vi "InitMessageBroker.vi"(8 "error in (no error)":errorcluster, 10 "Topic Actor":refnum<class "Topic Actor.lvclass">, 11 "Broker Name":string) -> (0 "error out":errorcluster, 3 "Message Broker Ref":refnum<data-value>)   [LabVIEW 2016, in "Stream Mediator.lvlib" / "Message Broker.lvclass"]
doc: "--\nCopyright © 2017 Composed SystemsI All rights reserved.\n\nAuthor: Jon McBee <jon.mcbee@composed.io>\n\nThis library is provided \"AS IS\" ,WITHOUT WARRANTIES OR\nCONDITIONS OF ANY KIND, either express or implied.\n\nComposed Systems -- composed.io\n\nStream 0.0.1.1\nJon McBee - Composed Systems\nCopyright (c) 2017, Composed Systems"
uses:
  <userlib>/Composed Systems/Stream/Mediator/Classes/Message Broker/Message Broker.lvclass
  <userlib>/Composed Systems/Stream/Mediator/Classes/Topic Actor/Topic Actor.lvclass
  <userlib>/Composed Systems/Stream/Mediator/Classes/Topic Actor Look Up Table/Topic Actor Look Up Table.lvclass
  <userlib>/Composed Systems/Stream/Mediator/Classes/Message Broker/Message Broker.lvclass/Message Broker.ctl
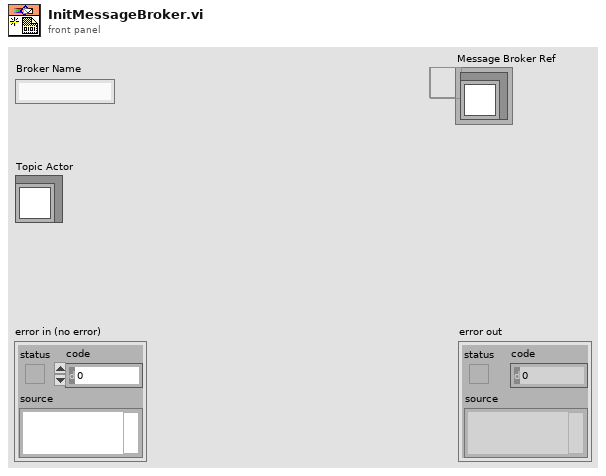
[diagram p1: front panel]
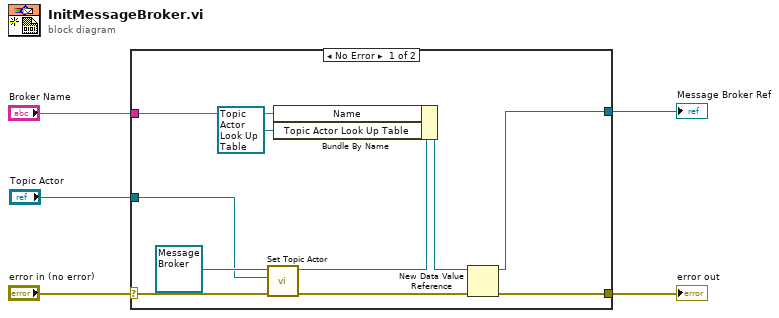
[diagram p0: block diagram]
diagram:
  n1 = case shown="No Error" "error in (no error)" {
    selector: "error in (no error)" -> [w8 w16]
    tunnel: [w15 w16] -> w4
    tunnel: [w14 _] -> w3
    tunnel: "Broker Name" -> [w11 _]
    tunnel: "Topic Actor" -> [w6 _]
    frame No Error {
      n2 = call-dynamic "Set Topic Actor.vi"("error in (no error)"=w8, "Topic Actor"=w6, "Message Broker in"=refnum<class "Message Broker.lvclass"> refnum ("Message Broker.lvclass")) -> ("error out"=w7:errorcluster, "Message Broker out"=w9:refnum<class "Message Broker.lvclass">)  [unwired: 7 in]
      n3 = Bundle By Name(cluster=w9, "Name"=w11, "Topic Actor Look Up Table"=refnum<class "Topic Actor Look Up Table.lvclass"> refnum) -> (w13:refnum<class "Message Broker.lvclass">)
      n4 = New Data Value Reference(data value=w13, error in=w7) -> (data value reference=w14:refnum<data-value>, error out=w15:errorcluster)
    }
    frame Error {
    }
  }
  "error out" <- w4
  "Message Broker Ref" <- w3
